vi "slider_outlet.vi"(9 "h02 (initial height of Tank 2)\n[m]":dbl, 10 "a2 (outlet of Tank 2)\n[m²]":dbl, 11 "Slide in":refnum<vi>) -> ()   [LabVIEW 2020]
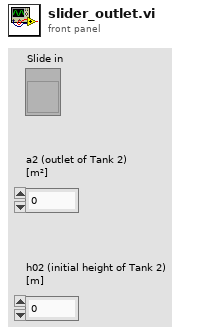
[diagram p1: front panel]
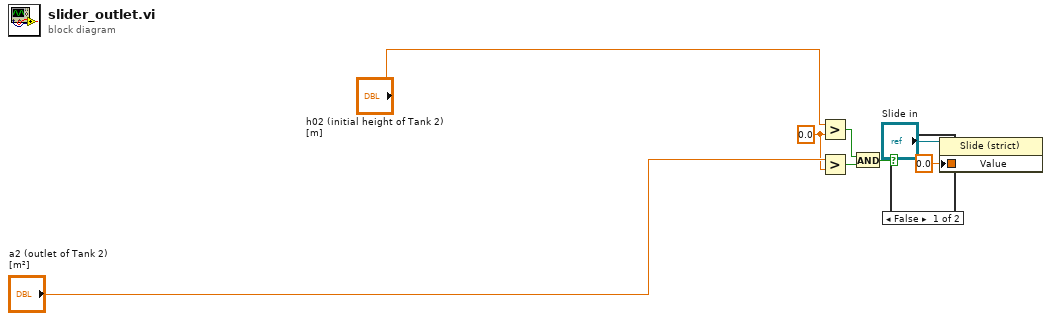
[diagram p0: block diagram]
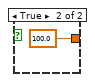
[diagram p2: hidden frame]
diagram:
  w6 = 0.0 ("y")
  n1 = Greater?(x="h02 (initial height of Tank 2)\n[m]", y=w6) -> (0:w2:bool)
  n2 = Greater?(x="a2 (outlet of Tank 2)\n[m²]", y=w6) -> (0:w3:bool)
  n3 = And(x=w2, y=w3) -> (x .and. y?=w4:bool)
  n4 = case shown="False" w4 {
    tunnel: [0.0 100.0 ("y")] -> w5
    frame False {
    }
    frame True {
    }
  }
  n5 = property on="Property Node" class="Slide (strict)"(reference="Slide in", "Value"=w5) -> ()  [unwired: 1 in, 2 out]
